vi "FPGA-no_chopper.vi"() -> ()   [LabVIEW 2009]
uses:
  Sequence.ctl
  Signal Options.ctl
  <vilib>/Platform/TimedLoop/XDataNode/XDataNode.xnode
  <vilib>/Platform/TimedLoop/XDataNode/loadlvalarms.vi
  <vilib>/Platform/TimedLoop/XDataNode/timing_clust.ctl
  <vilib>/Platform/TimedLoop/XDataNode/nitl_modes.ctl
  <vilib>/Platform/TimedLoop/XDataNode/wakeup.ctl
  <vilib>/eio/EIONode/EIONode.xnode
  <vilib>/rvi/eio/nirviEIOImplementation/nirviEIOImplementation.xnode
  <vilib>/rvi/eio/common/nirviEmuTemplateMethod_noerrors.vi
  <vilib>/rvi/eio/common/nirviEmuClasses.ctl
  <vilib>/Platform/TimedLoop/XDataNode/XDNodeRunTimeDep.lvlib
panel:
  in  "Squeezed AOM Signal 1+2 Sign":bool
  in  "Squeezed AOM Signal 2 start":u64
  in  "Squeezed AOM Signal 2 stop":u64
  in  "Trigger Phase Acquisition":bool
  in  "Phase Trigger Period":u32
  in  "Trigger Shot Aquisition":bool=TRUE
  in  "Shot Acquisiton Trigger Start":u64
  in  "Shot Acquisition Trigger Stop":u64
  in  "Memory Acquisition Trigger Stop":u64
  in  "WA Extra stop  6":u32
  in  "WA Extra start 6":u32
  in  "WA Extra stop  5":u32
  in  "WA Extra start 5":u32
  in  "WA Extra stop  4":u32
  in  "WA Extra start 4":u32
  in  "WA Extra stop  3":u32
  in  "WA Extra start 3":u32
  in  "WA Extra stop  2":u32
  in  "WA Extra start 2":u32
  in  "WA Extra start":u32
  in  "WA Extra stop":u32
  in  "WA Extra Sign":bool
  in  "WA Signal Switch 2 stop":u32
  in  "WA Signal Switch 2 start":u32
  in  "WA Signal Switch Sign":bool
  in  "WA Signal Switch stop":u32
  in  "WA Signal Switch start":u32
  in  "Squeezed AOM Signal Sign":bool
  in  "Squeezed AOM Control Sign":bool
  in  "Optical Density Sign":bool
  in  "SPME Gate 2 Sign":bool
  in  "SPME Gate 1 Sign":bool
  in  "SPME Signal Sign":bool
  in  "SPME Control Sign":bool
  in  "DLCZ Sign":bool
  in  "Raman Signal Sign":bool
  in  "Raman Control Sign":bool
  in  "Coherent Signal Sign":bool
  in  "WA Stop":bool
  in  "WA Trigger Output Sign":bool
  in  "WA Signal start":u32
  in  "WA Signal stop":u32
  in  "WA Signal Sign":bool
  in  "WA Repump start":u32
  in  "WA Repump stop":u32
  in  "WA Repump Sign":bool
  in  "WA Pump start":u32
  in  "WA Pump stop":u32
  in  "WA Pump Sign":bool
  in  "WA Control 2 - start":u32
  in  "WA Control 2 - stop":u32
  in  "WA Control 1 - start":u32
  in  "WA Control 1 - stop":u32
  in  "WA Control Sign":bool
  in  "WA Repetition Period":u32
  out "WA Active":bool
  in  "WA Trigger on Slope":enum8{"either", "false-true", "true-false"}(ring)=enum."true-false"
  out "WA Reset Interval":u64
  in  "WA Control Switch 2 - start":u32
  in  "WA Control Switch 2 - stop":u32
  in  "WA Control Switch 1 - start":u32
  in  "WA Control Switch 1 - stop":u32
  in  "WA Control Switch Sign":bool
  in  "Memory Acquisiton Trigger Start":u64
  in  "Memory Mode":bool
  out "Last N2":u64
  out "Last N1":u64
  in  "Desired Number of Trials":u64
  out "Number of Trials":u64
  out "Current N2":u64
  out "Current N1":u64
  in  "SPME Gate 2 - start":u64
  in  "SPME Gate 2 - stop":u64
  in  "SPME Gate 1 - start":u64
  in  "SPME Gate 1 - stop":u64
  out "SPME Count":u64
  out "Last SPME Interval between Resets":u64
  in  "SPME Period":u64
  in  "SPME Signal stop":u64
  in  "SPME Control - start":u64
  in  "Num of SPME Pulses per Mem Seq":u64=100
  in  "SPME Signal start":u64
  in  "SPME Control - stop":u64
  in  "SPME Start":u64
  in  "Raman/OD Acquisition Delay":u64
  in  "Squeezed AOM Signal 1 start":u64
  in  "Squeezed AOM Signal 1 stop":u64
  in  "Stop":bool
  out "Active":bool
  in  "Trapping Duration":u64
  in  "Pump Duration":u64
  in  "Repump Duration":u64
  out "Memory Timer":u64
  in  "Memory Mode":T1=enum."Coherent Memory Sequence"
  in  "Raman Control - stop":u64
  in  "Raman Control - start":u64
  in  "Raman Signal - stop":u64
  in  "Raman Signal - start":u64
  in  "Optical Density - start":u64
  in  "Optical Density - stop":u64
  in  "DLCZ width":u64
  in  "DLCZ Period":u32
  out "Last DLCZ Period":u64
  in  "DLCZ Stop":u64
  in  "DLCZ Start":u64
  in  "Control - start":u64
  in  "Control - stop":u64
  in  "Control Sign":bool
  out "Last Memory Period":u64
  in  "Coherent Signal start":u64
  in  "Coherent Signal stop":u64
  out "Global Time":u64
  in  "Output Trigger Sign":bool
  in  "Trigger on Slope":enum8{"either", "false-true", "true-false"}(ring)=enum."true-false"
  in  "Repetition Period":u32
  in  "Memory Sequence Duration":u64=240000
  out "Current State":T2
  out "Last Global Period":u64
  # "Alignment - Lights On"
  # "Corresponds to 5MHz by default"
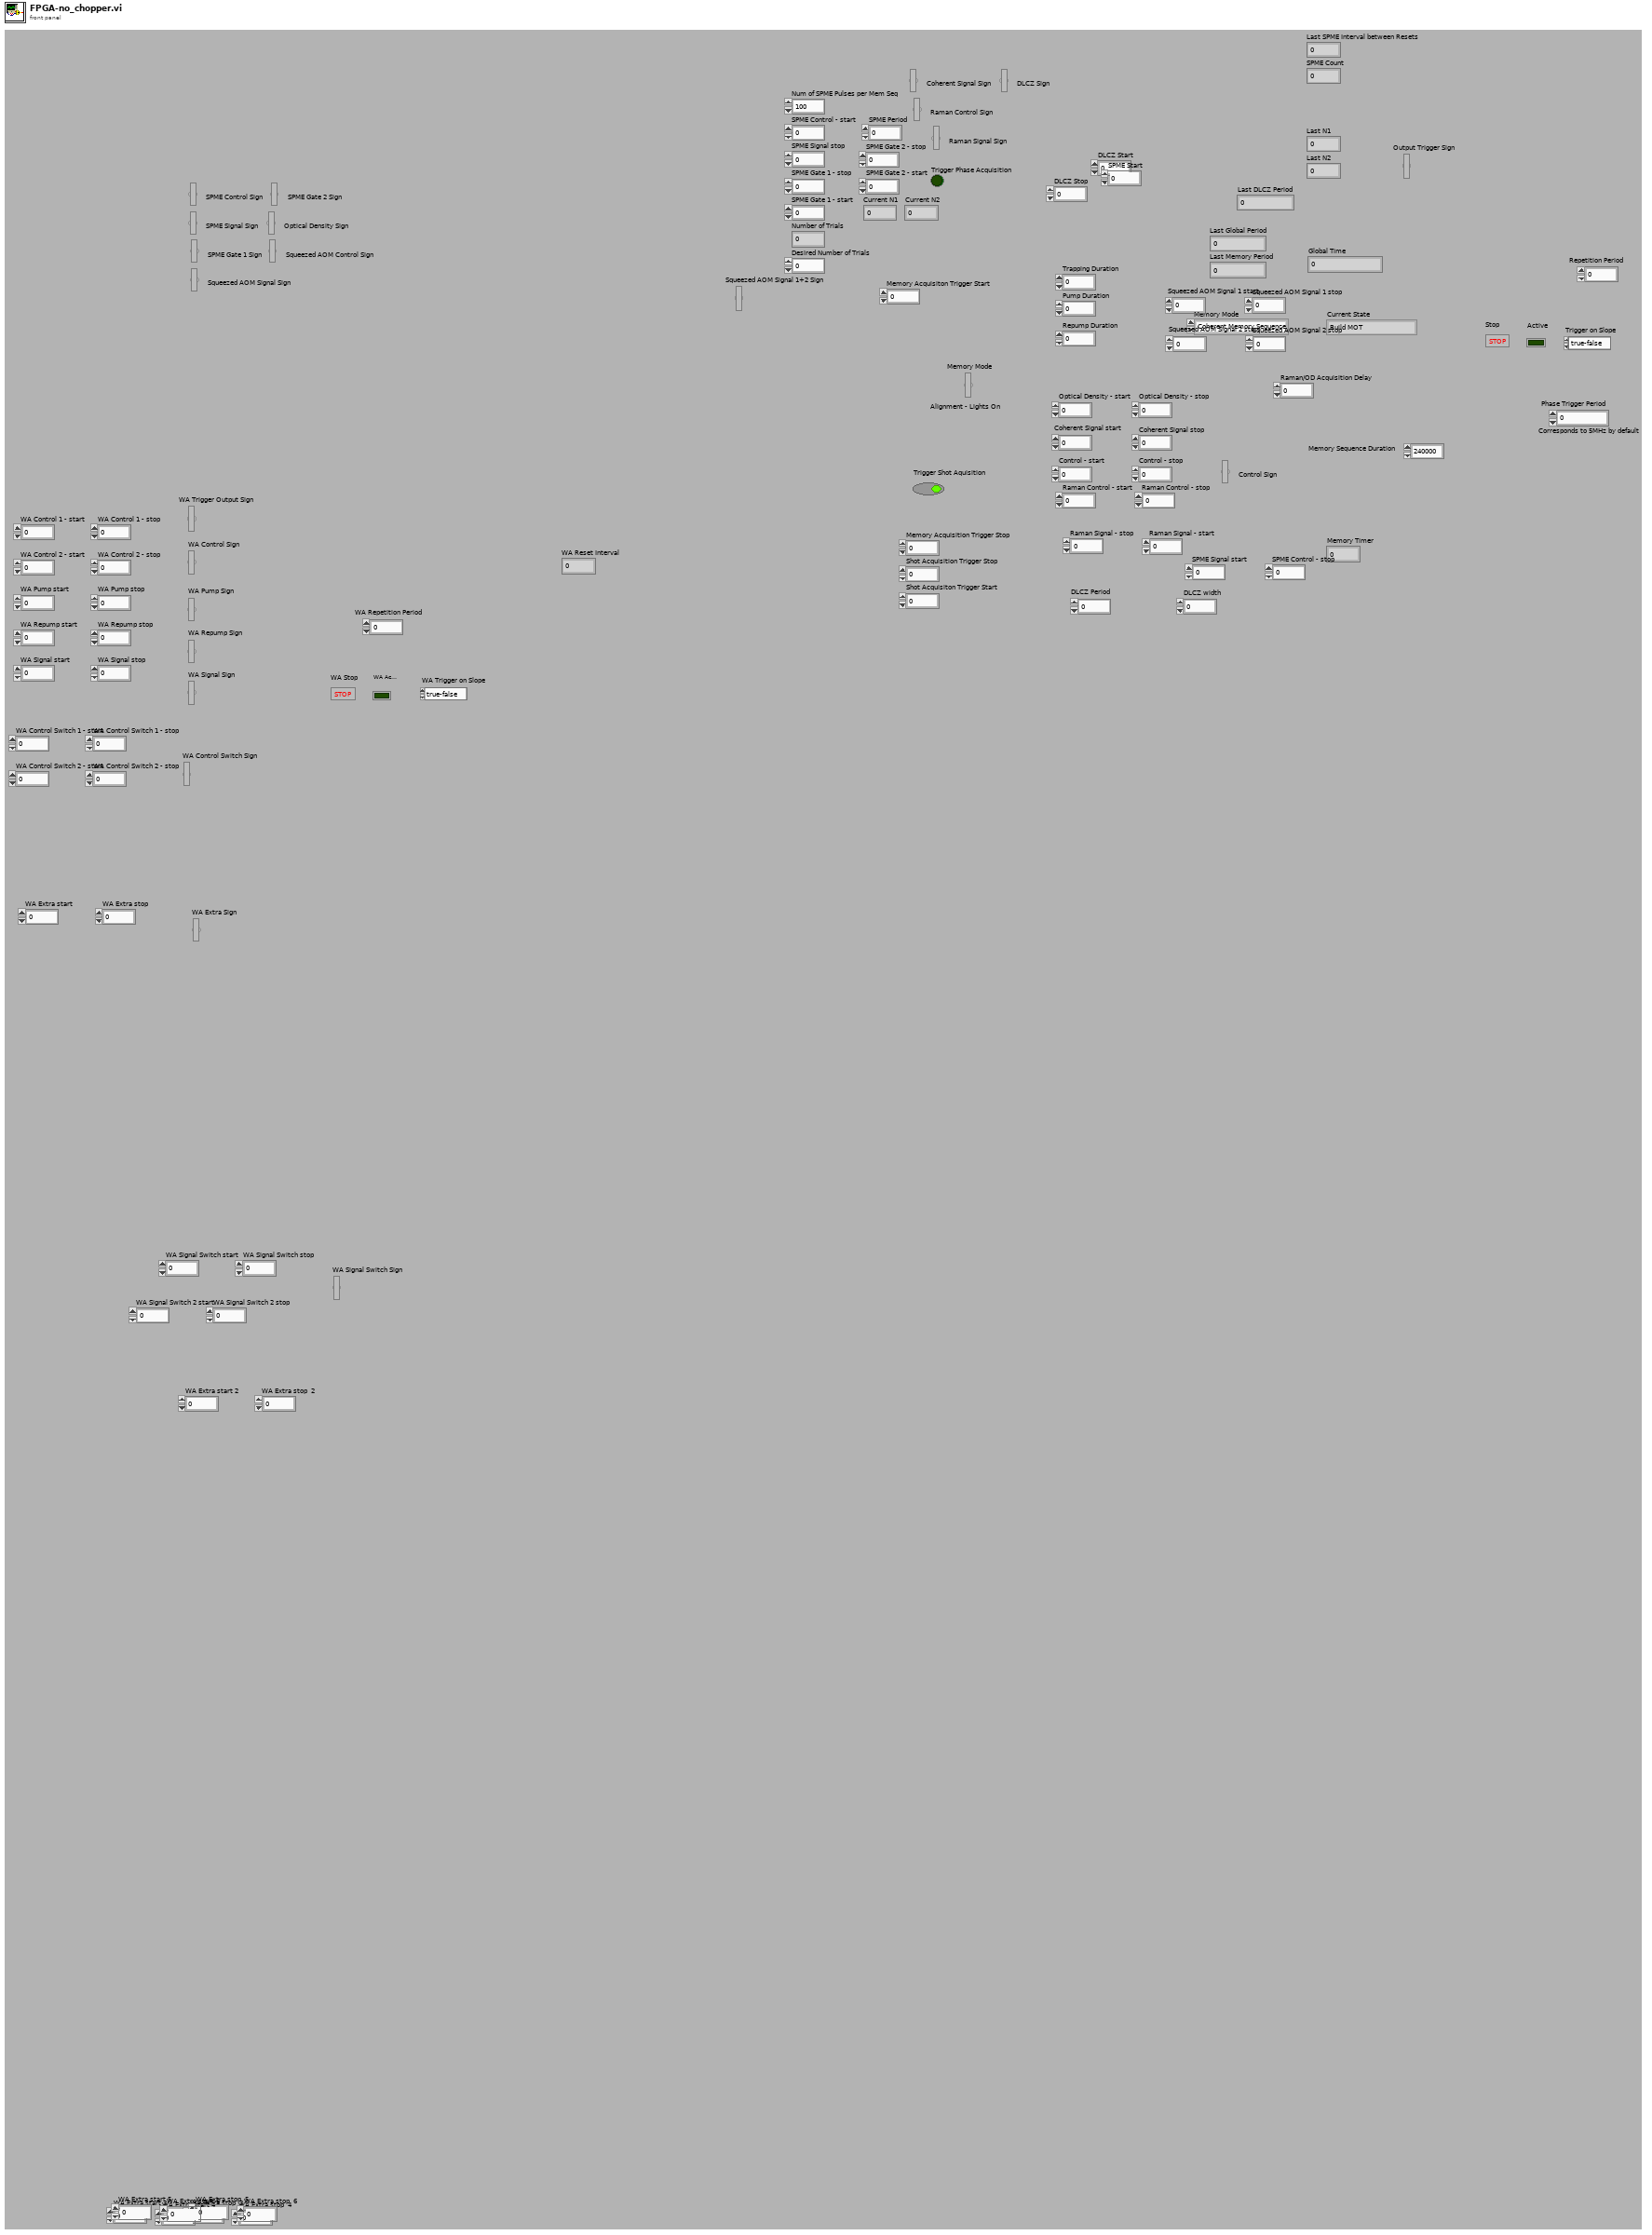
[diagram p1: front panel]
types:
  T1 = typedef "Signal Options.ctl" = enum16{"Cycle Trap - Standby", "Generate DLCZ Pulses", "Measure Optical Density", "Measure Raman", "Single Photon Memory Efficiency", "Coherent Memory Sequence", "Squeezed AOM Memory Sequence", "Squeezed Chopper Memory Sequence"}
  T2 = typedef "Sequence.ctl" = enum16{"Build MOT", "Memory Sequence", "Alignment - Lights On"}
  T3 = typedef "XDNodeRunTimeDep.lvlib/timing_clust.ctl" = cluster{"Expected End [f-1]":u64, "Actual End [f-1]":u64, "Finished Late? [f-1]":bool, "Expected End [i-1]":u64, "Actual End [i-1]":u64, "Finished Late? [i-1]":bool, "Expected Start [i]":u64, "Actual Start [i]":u64, "Expected Start [f]":u64, "Actual Start [f]":u64, "Source Name":string, "Structure Name":string, "Period":i64, "Deadline":i64, "Offset":i64, "Start":i64, "Priority":i32, "Timeout":i32, "Mode":T4, "Wakeup Reason":T5, "Error":errorcluster, "Source Type":string, "Secondary Source Type":string, "Global End Time":u64, "Global Start Time":u64, "Frame Duration":u64, "Iteration Duration":u64, "Assigned CPU":i32, "I/O Scan Engine Mode":u32}
  T4 = typedef "XDNodeRunTimeDep.lvlib/nitl_modes.ctl" = enum32{"No Change", "Process missed periods, maintain original phase", "Discard missed periods, maintain original phase", "Process missed periods, ignore original phase", "Discard missed periods, ignore original phase"}
  T5 = typedef "XDNodeRunTimeDep.lvlib/wakeup.ctl" = enum32{"Normal", "Aborted", "Asynchronous wakeup", "Timing source error", "Timed loop error", "Timeout"}
  T6 = typedef "nirviEmuClasses.ctl" = enum16{"IO Read", "IO Write", "Method", "Property Read", "Property Write"}
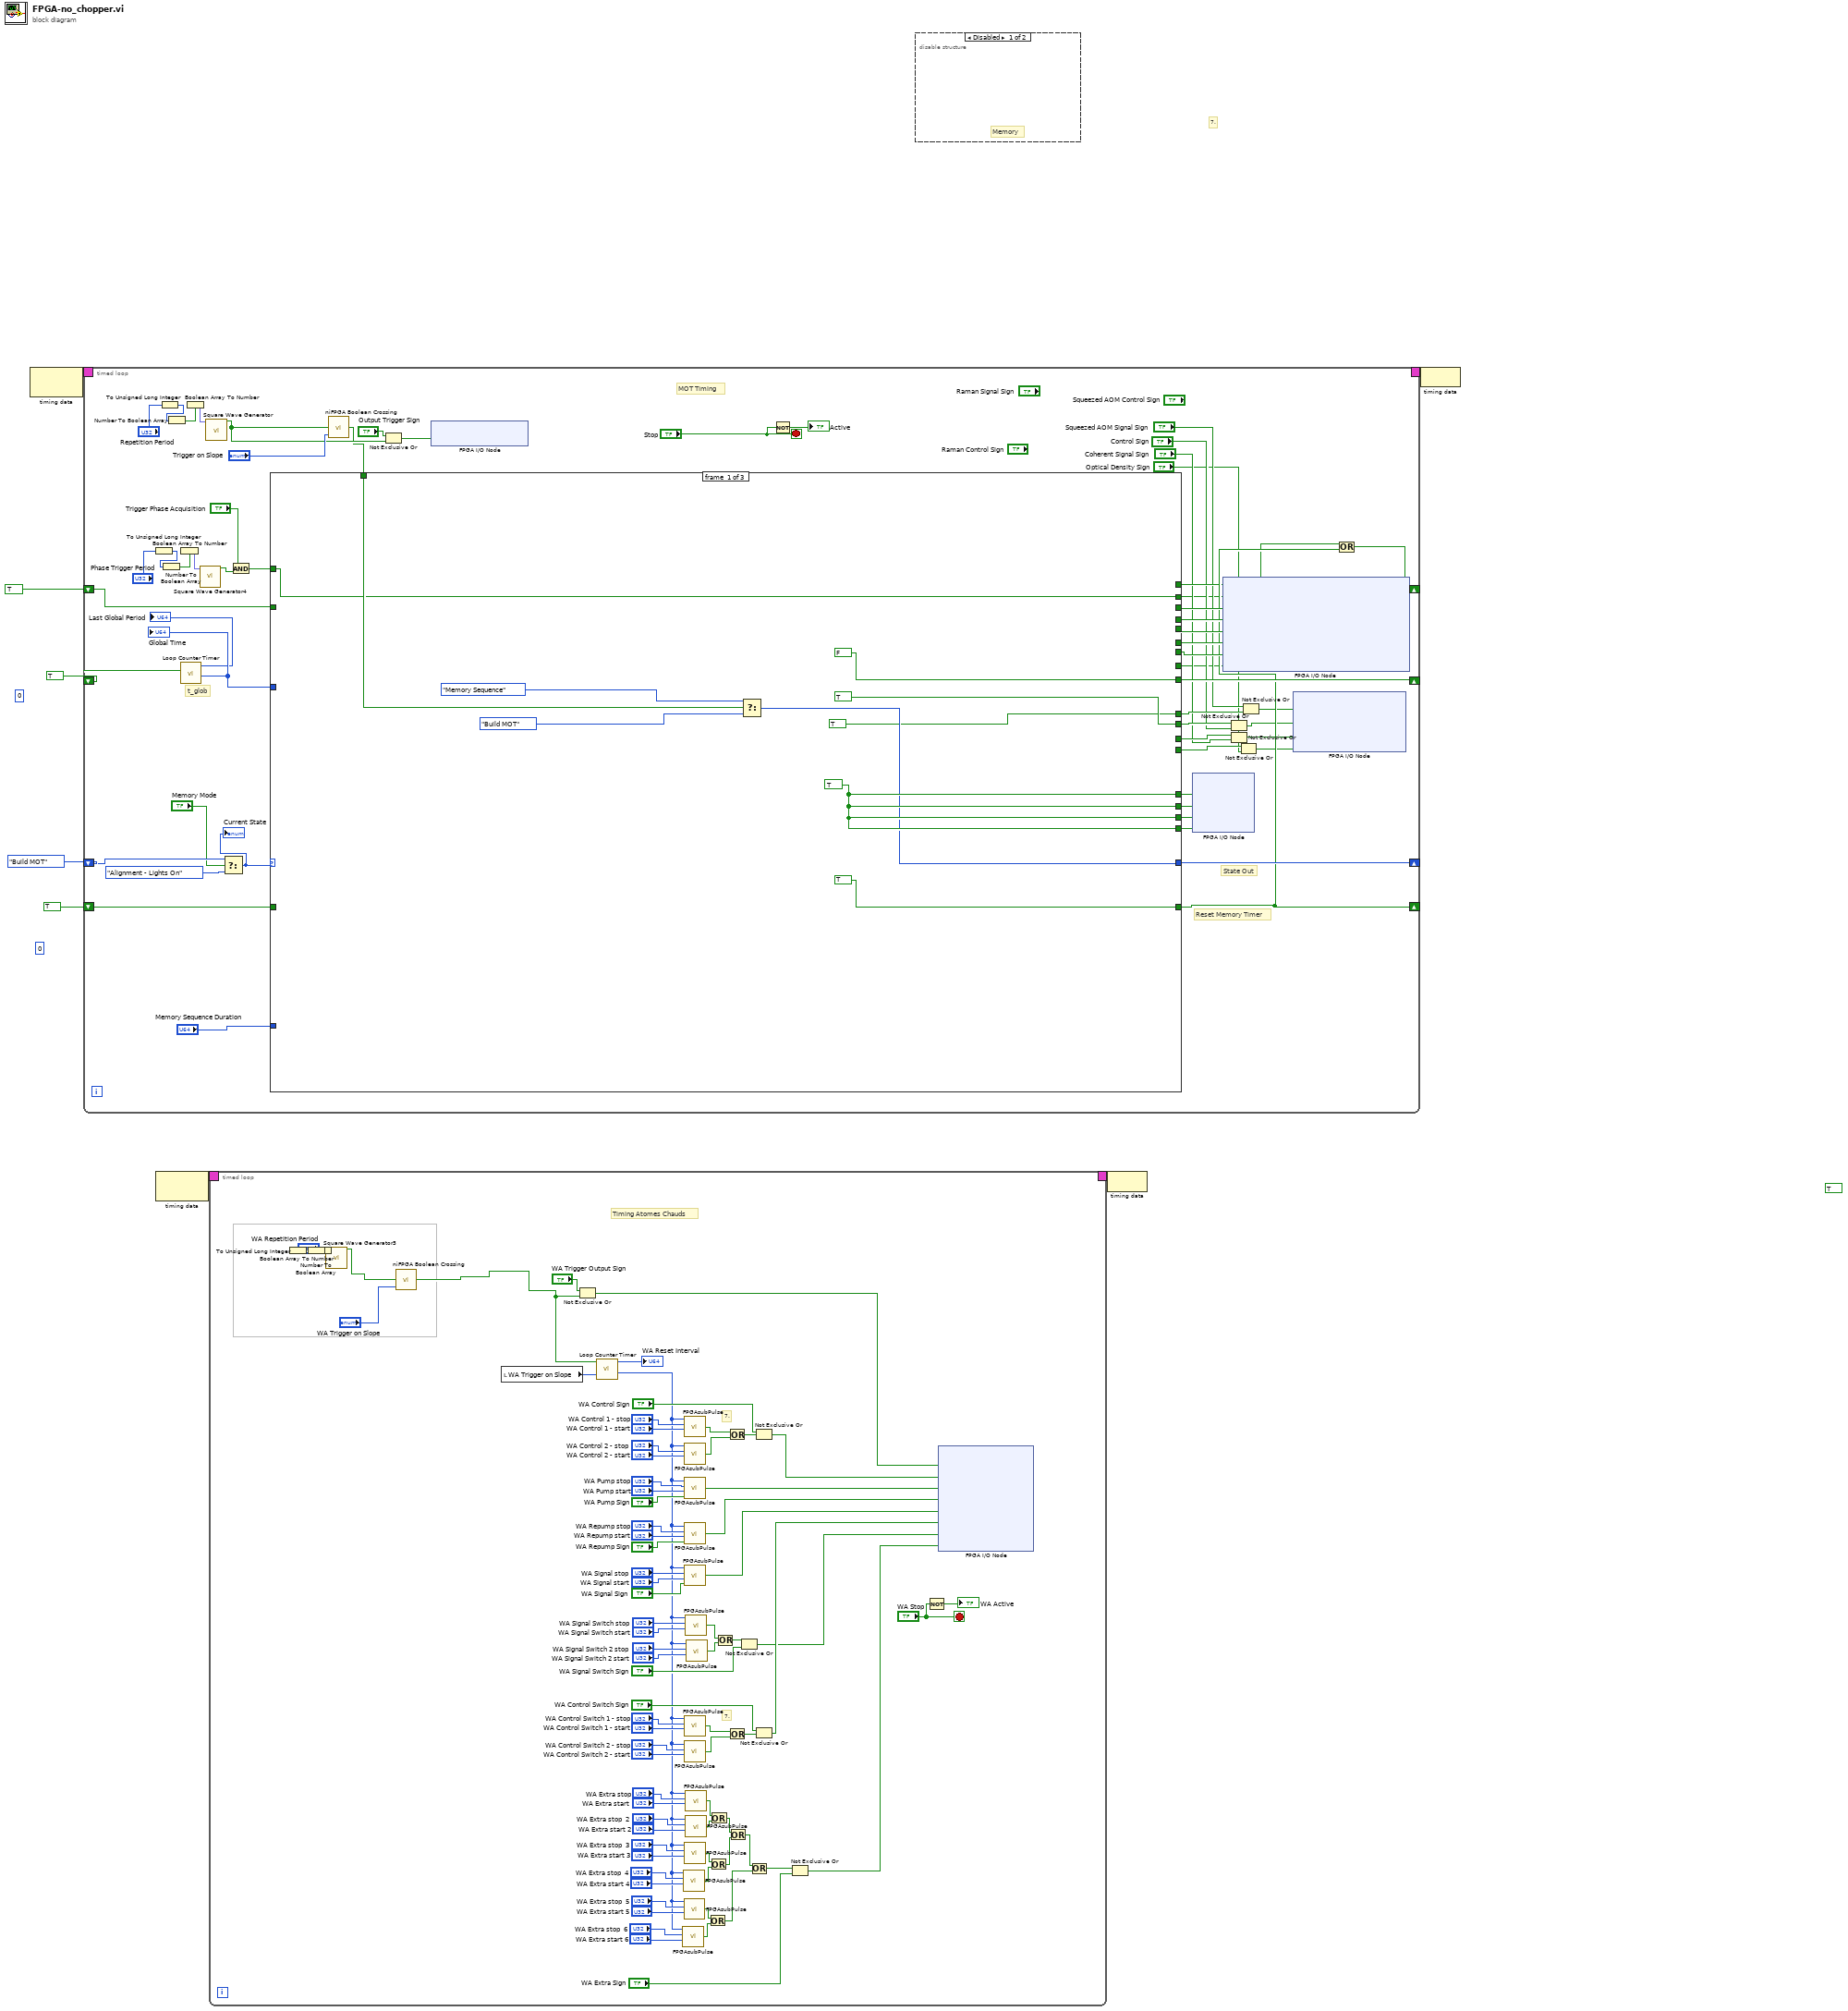
[diagram p0: block diagram]
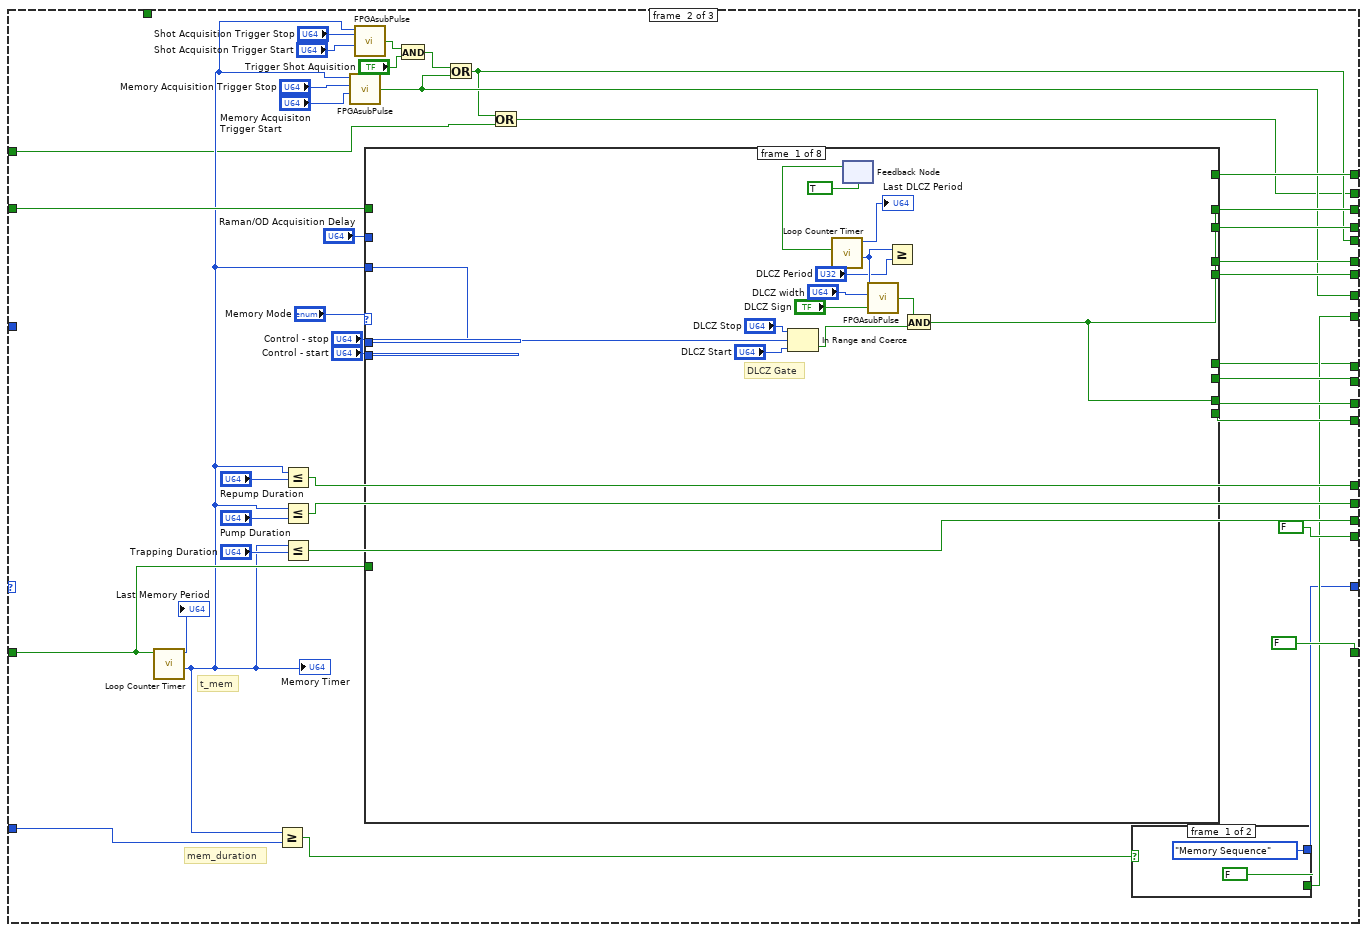
[diagram p3: hidden frame]
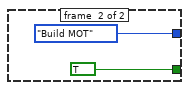
[diagram p4: hidden frame]
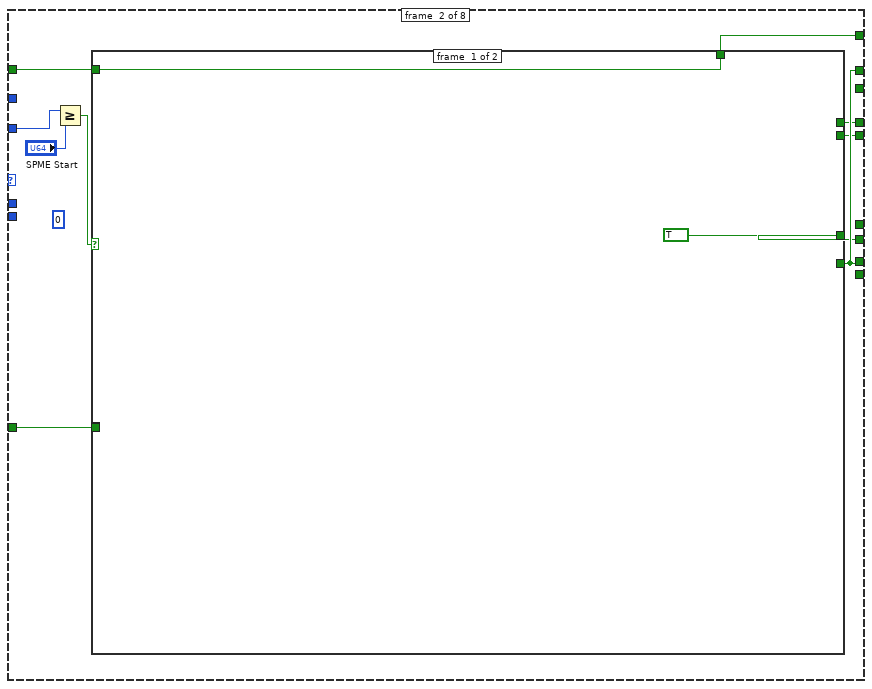
[diagram p5: hidden frame]
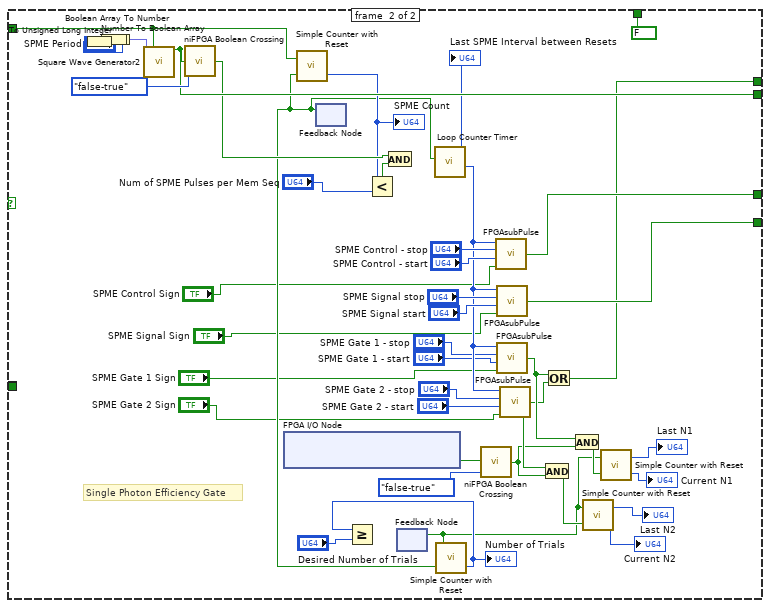
[diagram p6: hidden frame]
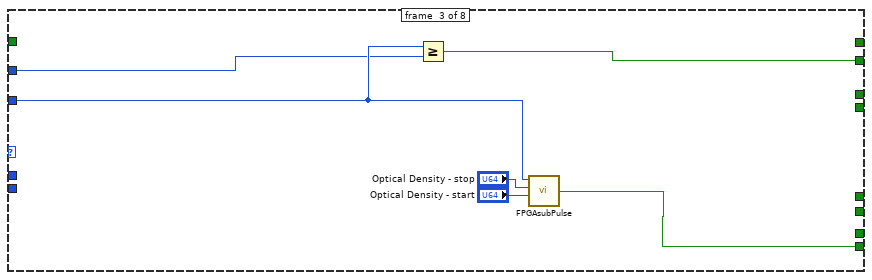
[diagram p7: hidden frame]
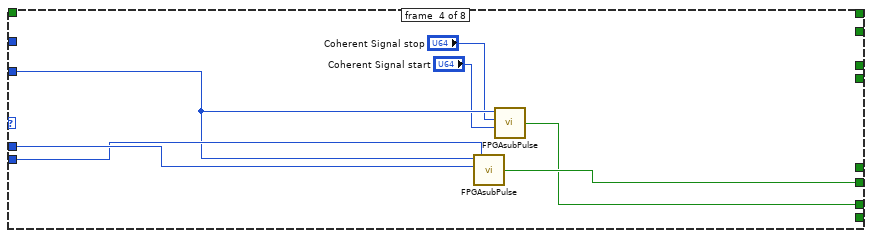
[diagram p8: hidden frame]
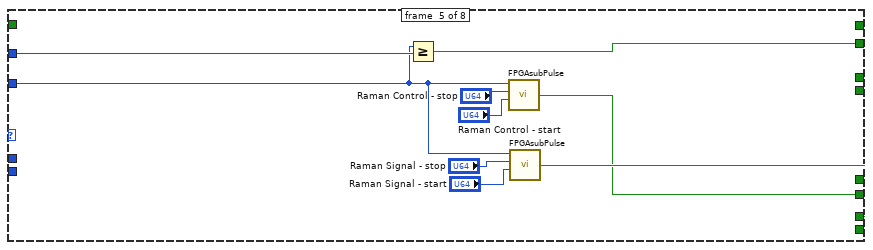
[diagram p9: hidden frame]
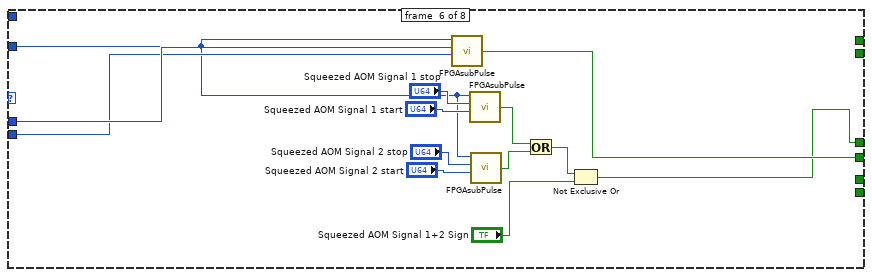
[diagram p10: hidden frame]
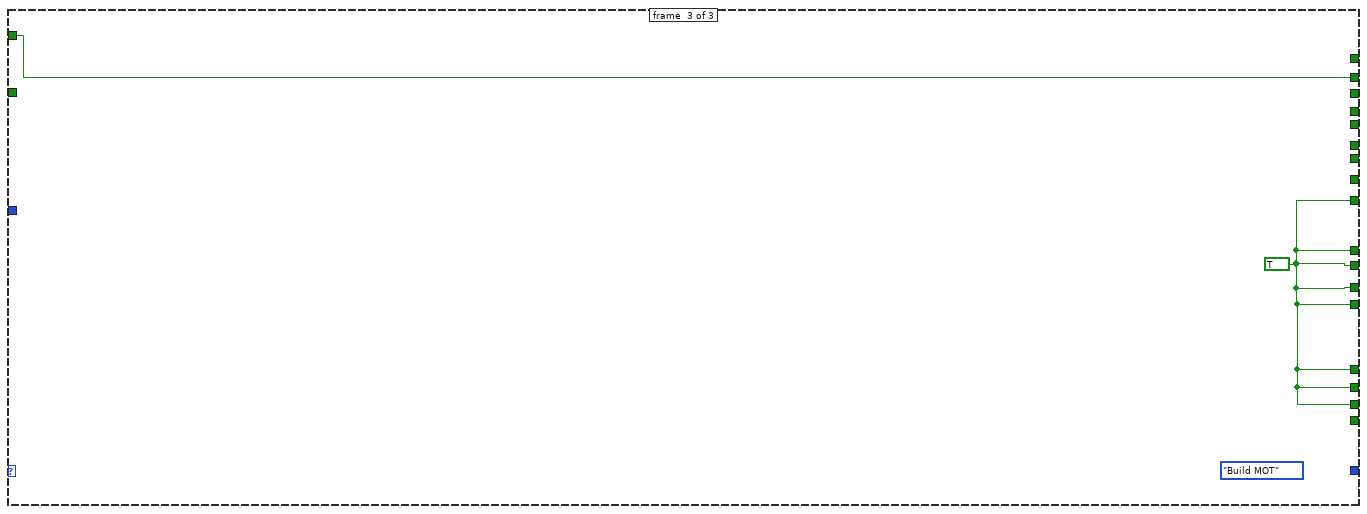
[diagram p13: hidden frame]
diagram:
  (unwired) u64 0
  (unwired) u64 0
  (unwired) TRUE
  # "7."
  n1 = node-c288() -> (w8:T3)  [unwired: 1 out]
  n2 = timed-loop {
    timing: w8 -> [_]
    timing-out: [_] -> w7
    shift-right: [w61] -> _
    shift-left: Sequence."Build MOT" ("Sequence") -> [w29]
    shift-right: [w43] -> _
    shift-left: TRUE -> [w54]
    shift-right: [w33] -> _
    shift-left: TRUE -> [w49]
    shift-right: [w31] -> _
    shift-left: TRUE -> [w32]
    stop <- "Stop" stop-if-true
    # "MOT Timing"
    # "Reset Memory Timer"
    # "State Out"
    # "t_glob"
    n3 = To Unsigned Long Integer(number="Phase Trigger Period") -> (unsigned 32bit integer=w12:u32)
    n4 = To Unsigned Long Integer(number="Repetition Period") -> (unsigned 32bit integer=w55:u32)
    n5 = Number To Boolean Array(number=w12) -> (Boolean array=w14:bool[])
    n6 = Number To Boolean Array(number=w55) -> (Boolean array=w57:bool[])
    n7 = Boolean Array To Number(Boolean array=w14) -> (number=w13:fxp<+,32,0>)
    n8 = call "Loop Counter Timer.vi"("Reset"=w54) -> ("Loop Counter"=w53:u64, "Last Interval between Resets"=→"Last Global Period":u64)  [unwired: 3 in, 2 out]
    "Global Time" <- w53
    n9 = Boolean Array To Number(Boolean array=w57) -> (number=w56:fxp<+,32,0>)
    n10 = call "Square Wave Generator4"("frequency (periods/tick)"=w13) -> ("square wave out"=w11:bool)  [unwired: 14 in]
    n11 = call "Square Wave Generator"("frequency (periods/tick)"=w56) -> ("square wave out"=w39:bool)  [unwired: 14 in]
    n12 = Select(t=w29, s="Memory Mode", f=Sequence."Alignment - Lights On" ("Sequence")) -> (s? t:f=w27:T2)
    "Current State" <- w27
    n13 = And(x="Trigger Phase Acquisition", y=w11) -> (x .and. y?=w9:bool)
    n14 = call <vilib>:"niFPGA Boolean Crossing.vi"("input"=w39, "direction"="Trigger on Slope") -> ("crossing"=w37:bool)  [unwired: 1 in, 6 out]
    n15 = case shown="\"Memory Sequence\"" w27 {
      tunnel: [w246 w272 _] -> w61
      tunnel: [w247 FALSE _] -> w62
      tunnel: [FALSE w273 w423] -> w43
      tunnel: w53 -> [_ _ _]
      tunnel: [w247 w283 w423] -> w52
      tunnel: [w247 w284 w423] -> w51
      tunnel: [w247 w285 w423] -> w50
      tunnel: [TRUE FALSE _] -> w33
      tunnel: w49 -> [_ w265 _]
      tunnel: "Memory Sequence Duration" -> [_ w289 _]
      tunnel: [TRUE ("Boolean") w281 w423] -> w47
      tunnel: [_ w280 w423] -> w46
      tunnel: [_ w279 w423] -> w45
      tunnel: [_ w271 _] -> w42
      tunnel: [_ w269 _] -> w41
      tunnel: [TRUE ("Boolean") w270 w423] -> w40
      tunnel: w37 -> [w245 _ _]
      tunnel: [_ w253 _] -> w36
      tunnel: [_ w267 _] -> w35
      tunnel: [_ w266 _] -> w34
      tunnel: w32 -> [_ w264 _]
      tunnel: [_ w263 _] -> w30
      tunnel: [_ w254 _] -> w17
      tunnel: [w241 w252 w422] -> w16
      tunnel: w9 -> [w241 w251 w422]
      frame #0 {
        w247 = TRUE
        n16 = Select(t=Sequence."Memory Sequence" ("Sequence"), s=w245, f=Sequence."Build MOT" ("Sequence")) -> (s? t:f=w246:T2)
      }
      frame #1 {
        # "mem_duration"
        # "t_mem"
        n17 = call "Loop Counter Timer.vi"("Reset"=w265) -> ("Loop Counter"=w258:u64, "Last Interval between Resets"=→"Last Memory Period":u64)  [unwired: 3 in, 2 out]
        "Memory Timer" <- w258
        n18 = Greater Or Equal?(x=w258, y=w289) -> (x >= y?=w274:bool)
        n19 = Less Or Equal?(x=w258, y="Repump Duration") -> (x <= y?=w283:bool)
        n20 = Less Or Equal?(x=w258, y="Pump Duration") -> (x <= y?=w284:bool)
        n21 = Less Or Equal?(x=w258, y="Trapping Duration") -> (x <= y?=w285:bool)
        n22 = call "FPGAsubPulse.vi"("Signal start"="Memory Acquisiton Trigger Start", "Signal stop"="Memory Acquisition Trigger Stop", "Clock"=w258) -> ("Boolean"=w254:bool)  [unwired: 1 in]
        n23 = call "FPGAsubPulse.vi"("Signal start"="Shot Acquisiton Trigger Start", "Signal stop"="Shot Acquisition Trigger Stop", "Clock"=w258) -> ("Boolean"=w257:bool)  [unwired: 1 in]
        n24 = case shown="\"Squeezed AOM Memory Sequence\"" "Memory Mode" {
          tunnel: w258 -> [w300 w318 w389 w397 w401 w414 _ _]
          tunnel: [_ w314 _ w396 w403 w419 _ _] -> w281
          tunnel: [_ _ w390 _ _ _ _ _] -> w280
          tunnel: [w296 w315 _ w395 w408 _ _ _] -> w279
          tunnel: "Control - stop" -> [_ _ _ w399 _ w421 _ _]
          tunnel: "Control - start" -> [_ _ _ w398 _ w420 _ _]
          tunnel: [_ _ w387 _ w400 _ _ _] -> w271
          tunnel: [w296 w315 _ _ _ _ _ _] -> w269
          tunnel: [_ _ _ _ _ w410 _ _] -> w270
          tunnel: "Raman/OD Acquisition Delay" -> [_ _ w388 _ w402 _ _ _]
          tunnel: [_ w313 _ _ _ _ _ _] -> w267
          tunnel: [_ w312 _ _ _ _ _ _] -> w266
          tunnel: w265 -> [_ w311 _ _ _ _ _ _]
          tunnel: w264 -> [_ w310 _ _ _ _ _ _]
          tunnel: [_ w309 _ _ _ _ _ _] -> w263
          frame #0 {
            # "DLCZ Gate"
            n25 = In Range and Coerce(upper limit="DLCZ Stop", x=w300, lower limit="DLCZ Start") -> (In Range?=w301:bool)  [unwired: 1 out]
            n26 = feedback #1(TRUE) -> (w306:bool)
            n27 = call "Loop Counter Timer.vi"("Reset"=w306) -> ("Loop Counter"=w304:u64, "Last Interval between Resets"=→"Last DLCZ Period":u64)  [unwired: 3 in, 2 out]
            n28 = call "FPGAsubPulse.vi"("Signal Sign"="DLCZ Sign", "Signal stop"="DLCZ width", "Clock"=w304) -> ("Boolean"=w297:bool)  [unwired: 1 in]
            n29 = Greater Or Equal?(x=w304, y="DLCZ Period") -> (x >= y?=w307:bool)
            n30 = And(x=w297, y=w301) -> (x .and. y?=w296:bool)
          }
          frame #1 {
            (unwired) u64 0
            n31 = Greater Or Equal?(x=w318, y="SPME Start") -> (x >= y?=w316:bool)
            n32 = case shown="False" w316 {
              tunnel: [_ w352] -> w315
              tunnel: [TRUE ("Boolean") w367] -> w314
              tunnel: [_ w356] -> w313
              tunnel: [_ w346] -> w312
              tunnel: [_ w355] -> _
              tunnel: w311 -> [_ w355]
              tunnel: w310 -> [w319 w331]
              tunnel: [w319 FALSE] -> w309
              frame #0 {
              }
              frame #1 {
                # "Single Photon Efficiency Gate"
                n33 = To Unsigned Long Integer(number="SPME Period") -> (unsigned 32bit integer=w365:u32)
                n34 = Number To Boolean Array(number=w365) -> (Boolean array=w364:bool[])
                n35 = Boolean Array To Number(Boolean array=w364) -> (number=w363:fxp<+,32,0>)
                n36 = call "Square Wave Generator2"("frequency (periods/tick)"=w363, "reset"=w331) -> ("square wave out"=w356:bool)  [unwired: 13 in]
                n37 = call <vilib>:"niFPGA Boolean Crossing.vi"("input"=w356, "direction"=enum8{"either", "false-true", "true-false"}."false-true") -> ("crossing"=w332:bool)  [unwired: 1 in, 6 out]
                n38 = xnode "FPGA I/O Node"() -> ("SPME APD Counter Input"=w339:bool)  [unwired: 1 in, 1 out]
                n39 = feedback #2() -> (w328:bool)  [unwired: 1 in]
                n40 = call "Simple Counter with Reset.vi"("Add"=w328, "Reset"=w331) -> ("Loop Counter"=w330:u64)  [unwired: 1 out]
                "SPME Count" <- w330
                n41 = Less?(x=w330, y="Num of SPME Pulses per Mem Seq") -> (x < y?=w361:bool)
                n42 = And(x=w332, y=w361) -> (x .and. y?=w329:bool)
                n43 = feedback #3() -> (w333:bool)  [unwired: 1 in]
                n44 = call "Loop Counter Timer.vi"("Reset"=w328) -> ("Loop Counter"=w351:u64, "Last Interval between Resets"=→"Last SPME Interval between Resets":u64)  [unwired: 3 in, 2 out]
                n45 = call "Simple Counter with Reset.vi"("Add"=w328, "Reset"=w333) -> ("Loop Counter"=w341:u64)  [unwired: 1 out]
                "Number of Trials" <- w341
                n46 = Greater Or Equal?(x=w341, y="Desired Number of Trials") -> (x >= y?=w340:bool)
                n47 = call <vilib>:"niFPGA Boolean Crossing.vi"("input"=w339, "direction"=enum8{"either", "false-true", "true-false"}."false-true") -> ("crossing"=w338:bool)  [unwired: 1 in, 6 out]
                n48 = call "FPGAsubPulse.vi"("Signal Sign"="SPME Control Sign", "Signal start"="SPME Control - start", "Signal stop"="SPME Control - stop", "Clock"=w351) -> ("Boolean"=w367:bool)
                n49 = call "FPGAsubPulse.vi"("Signal Sign"="SPME Signal Sign", "Signal start"="SPME Signal start", "Signal stop"="SPME Signal stop", "Clock"=w351) -> ("Boolean"=w352:bool)
                n50 = call "FPGAsubPulse.vi"("Signal Sign"="SPME Gate 1 Sign", "Signal start"="SPME Gate 1 - start", "Signal stop"="SPME Gate 1 - stop", "Clock"=w351) -> ("Boolean"=w343:bool)
                n51 = call "FPGAsubPulse.vi"("Signal Sign"="SPME Gate 2 Sign", "Signal start"="SPME Gate 2 - start", "Signal stop"="SPME Gate 2 - stop", "Clock"=w351) -> ("Boolean"=w342:bool)
                n52 = And(x=w342, y=w338) -> (x .and. y?=w336:bool)
                n53 = Or(x=w343, y=w342) -> (x .or. y?=w346:bool)
                n54 = And(x=w343, y=w338) -> (x .and. y?=w335:bool)
                n55 = call "Simple Counter with Reset.vi"("Add"=w336, "Reset"=w333) -> ("Loop Counter"=→"Current N2":u64, "Last Count Before Reset"=→"Last N2":u64)
                n56 = call "Simple Counter with Reset.vi"("Add"=w335, "Reset"=w333) -> ("Loop Counter"=→"Current N1":u64, "Last Count Before Reset"=→"Last N1":u64)
              }
            }
          }
          frame #2 {
            n57 = Greater Or Equal?(x=w389, y=w388) -> (x >= y?=w387:bool)
            n58 = call "FPGAsubPulse.vi"("Signal start"="Optical Density - start", "Signal stop"="Optical Density - stop", "Clock"=w389) -> ("Boolean"=w390:bool)  [unwired: 1 in]
          }
          frame #3 {
            n59 = call "FPGAsubPulse.vi"("Signal start"=w398, "Signal stop"=w399, "Clock"=w397) -> ("Boolean"=w396:bool)  [unwired: 1 in]
            n60 = call "FPGAsubPulse.vi"("Signal start"="Coherent Signal start", "Signal stop"="Coherent Signal stop", "Clock"=w397) -> ("Boolean"=w395:bool)  [unwired: 1 in]
          }
          frame #4 {
            n61 = Greater Or Equal?(x=w401, y=w402) -> (x >= y?=w400:bool)
            n62 = call "FPGAsubPulse.vi"("Signal start"="Raman Control - start", "Signal stop"="Raman Control - stop", "Clock"=w401) -> ("Boolean"=w403:bool)  [unwired: 1 in]
            n63 = call "FPGAsubPulse.vi"("Signal start"="Raman Signal - start", "Signal stop"="Raman Signal - stop", "Clock"=w401) -> ("Boolean"=w408:bool)  [unwired: 1 in]
          }
          frame #5 {
            n64 = call "FPGAsubPulse.vi"("Signal start"=w420, "Signal stop"=w421, "Clock"=w414) -> ("Boolean"=w419:bool)  [unwired: 1 in]
            n65 = call "FPGAsubPulse.vi"("Signal start"="Squeezed AOM Signal 1 start", "Signal stop"="Squeezed AOM Signal 1 stop", "Clock"=w414) -> ("Boolean"=w412:bool)  [unwired: 1 in]
            n66 = call "FPGAsubPulse.vi"("Signal start"="Squeezed AOM Signal 2 start", "Signal stop"="Squeezed AOM Signal 2 stop", "Clock"=w414) -> ("Boolean"=w413:bool)  [unwired: 1 in]
            n67 = Or(x=w412, y=w413) -> (x .or. y?=w411:bool)
            n68 = Not Exclusive Or(1:"Squeezed AOM Signal 1+2 Sign", 2:w411) -> (0:w410:bool)
          }
          frame #6 {
          }
          frame #7 {
          }
        }
        n69 = And(x=w257, y="Trigger Shot Aquisition") -> (x .and. y?=w256:bool)
        n70 = Or(x=w256, y=w254) -> (x .or. y?=w253:bool)
        n71 = Or(x=w253, y=w251) -> (x .or. y?=w252:bool)
        n72 = case shown="True" w274 {
          tunnel: [FALSE TRUE] -> w273
          tunnel: [Sequence."Memory Sequence" ("Sequence") Sequence."Build MOT" ("Sequence")] -> w272
          frame #0 {
          }
          frame #1 {
          }
        }
      }
      frame #2 {
        (unwired) Sequence."Build MOT" ("Sequence")
        w423 = TRUE ("Boolean")
      }
    }
    n73 = Not Exclusive Or(1:w39, 2:"Output Trigger Sign") -> (0:w38:bool)
    n74 = xnode "FPGA I/O Node"("Experiment Trigger"=w38) -> ()  [unwired: 1 in, 1 out]
    n75 = Not(x="Stop") -> (.not. x?=→"Active":bool)
    n76 = xnode "FPGA I/O Node"("Repump"=w52, "Pump"=w51, "Trapping"=w50, "B-Field"=w62) -> ()  [unwired: 4 in, 4 out]
    n77 = xnode "FPGA I/O Node"("Memory-Shot-Phase Acquisition Trigger"=w16, "APD1 Gate"=w41, "Raman/Optical Density Acquisition Trigger"=w42, "Memory-Shot Aquisition Trigger"=w36, "Single Photon Memory Gate"=w34, "SPME Timer"=w35, "Memory Only Acquisition Trigger  for Phase"=w17) -> ()  [unwired: 7 in, 7 out]
    n78 = Not Exclusive Or(1:"Control Sign", 2:w47) -> (0:w23:bool)
    n79 = Not Exclusive Or(1:"Coherent Signal Sign", 2:w45) -> (0:w21:bool)
    n80 = Not Exclusive Or(1:"Optical Density Sign", 2:w46) -> (0:w19:bool)
    n81 = Not Exclusive Or(1:w40, 2:"Squeezed AOM Signal Sign") -> (0:w25:bool)
    n82 = xnode "FPGA I/O Node"("Pulsed Squeezing AOM"=w25, "Control"=w23, "Signal"=w21, "Optical Density"=w19) -> ()  [unwired: 4 in, 4 out]
    n83 = Or(x=w30, y=w33) -> (x .or. y?=w31:bool)
  }
  n84 = node-c288() -> (w2:T3)  [unwired: 1 out]
  n85 = timed-loop {
    timing: w2 -> [_]
    timing-out: [_] -> w1
    stop <- "WA Stop" stop-if-true
    # "Timing Atomes Chauds"
    # "7."
    # "7."
    n86 = To Unsigned Long Integer(number="WA Repetition Period") -> (unsigned 32bit integer=w465:u32)
    n87 = Number To Boolean Array(number=w465) -> (Boolean array=w463:bool[])
    n88 = Boolean Array To Number(Boolean array=w463) -> (number=w464:fxp<+,32,0>)
    n89 = call "Square Wave Generator3"("frequency (periods/tick)"=w464) -> ("square wave out"=w461:bool)  [unwired: 14 in]
    n90 = call <vilib>:"niFPGA Boolean Crossing.vi"("input"=w461, "direction"="WA Trigger on Slope") -> ("crossing"=w462:bool)  [unwired: 1 in, 6 out]
    n91 = local read "WA Trigger on Slope"() -> (w480:enum8{"either", "false-true", "true-false"})
    n92 = Not Exclusive Or(1:w462, 2:"WA Trigger Output Sign") -> (0:w479:bool)
    n93 = call "Loop Counter Timer.vi"("Trigger Direction"=w480, "Waveform"=w462) -> ("Loop Counter"=w429:u64, "Last Interval between Resets"=→"WA Reset Interval":u64)  [unwired: 2 in, 2 out]
    n94 = call "FPGAsubPulse.vi"("Signal start"="WA Extra start 6", "Signal stop"="WA Extra stop  6", "Clock"=w429) -> ("Boolean"=w430:bool)  [unwired: 1 in]
    n95 = call "FPGAsubPulse.vi"("Signal start"="WA Extra start 4", "Signal stop"="WA Extra stop  4", "Clock"=w429) -> ("Boolean"=w436:bool)  [unwired: 1 in]
    n96 = call "FPGAsubPulse.vi"("Signal start"="WA Extra start 5", "Signal stop"="WA Extra stop  5", "Clock"=w429) -> ("Boolean"=w431:bool)  [unwired: 1 in]
    n97 = call "FPGAsubPulse.vi"("Signal start"="WA Control 1 - start", "Signal stop"="WA Control 1 - stop", "Clock"=w429) -> ("Boolean"=w489:bool)  [unwired: 1 in]
    n98 = call "FPGAsubPulse.vi"("Signal start"="WA Control 2 - start", "Signal stop"="WA Control 2 - stop", "Clock"=w429) -> ("Boolean"=w488:bool)  [unwired: 1 in]
    n99 = call "FPGAsubPulse.vi"("Signal Sign"="WA Pump Sign", "Signal start"="WA Pump start", "Signal stop"="WA Pump stop", "Clock"=w429) -> ("Boolean"=w477:bool)
    n100 = call "FPGAsubPulse.vi"("Signal Sign"="WA Repump Sign", "Signal start"="WA Repump start", "Signal stop"="WA Repump stop", "Clock"=w429) -> ("Boolean"=w476:bool)
    n101 = call "FPGAsubPulse.vi"("Signal Sign"="WA Signal Sign", "Signal start"="WA Signal start", "Signal stop"="WA Signal stop", "Clock"=w429) -> ("Boolean"=w475:bool)
    n102 = call "FPGAsubPulse.vi"("Signal start"="WA Control Switch 1 - start", "Signal stop"="WA Control Switch 1 - stop", "Clock"=w429) -> ("Boolean"=w471:bool)  [unwired: 1 in]
    n103 = call "FPGAsubPulse.vi"("Signal start"="WA Control Switch 2 - start", "Signal stop"="WA Control Switch 2 - stop", "Clock"=w429) -> ("Boolean"=w472:bool)  [unwired: 1 in]
    n104 = call "FPGAsubPulse.vi"("Signal start"="WA Extra start 3", "Signal stop"="WA Extra stop  3", "Clock"=w429) -> ("Boolean"=w439:bool)  [unwired: 1 in]
    n105 = call "FPGAsubPulse.vi"("Signal start"="WA Signal Switch start", "Signal stop"="WA Signal Switch stop", "Clock"=w429) -> ("Boolean"=w456:bool)  [unwired: 1 in]
    n106 = call "FPGAsubPulse.vi"("Signal start"="WA Extra start", "Signal stop"="WA Extra stop", "Clock"=w429) -> ("Boolean"=w447:bool)  [unwired: 1 in]
    n107 = call "FPGAsubPulse.vi"("Signal start"="WA Extra start 2", "Signal stop"="WA Extra stop  2", "Clock"=w429) -> ("Boolean"=w446:bool)  [unwired: 1 in]
    n108 = call "FPGAsubPulse.vi"("Signal start"="WA Signal Switch 2 start", "Signal stop"="WA Signal Switch 2 stop", "Clock"=w429) -> ("Boolean"=w455:bool)  [unwired: 1 in]
    n109 = Or(x=w431, y=w430) -> (x .or. y?=w427:bool)
    n110 = Or(x=w439, y=w436) -> (x .or. y?=w438:bool)
    n111 = Or(x=w447, y=w446) -> (x .or. y?=w437:bool)
    n112 = Or(x=w456, y=w455) -> (x .or. y?=w452:bool)
    n113 = Or(x=w489, y=w488) -> (x .or. y?=w484:bool)
    n114 = Or(x=w471, y=w472) -> (x .or. y?=w473:bool)
    n115 = Or(x=w437, y=w438) -> (x .or. y?=w428:bool)
    n116 = Not Exclusive Or(1:"WA Signal Switch Sign", 2:w452) -> (0:w451:bool)
    n117 = Or(x=w428, y=w427) -> (x .or. y?=w426:bool)
    n118 = Not Exclusive Or(1:w484, 2:"WA Control Sign") -> (0:w478:bool)
    n119 = Not Exclusive Or(1:w473, 2:"WA Control Switch Sign") -> (0:w466:bool)
    n120 = Not Exclusive Or(1:"WA Extra Sign", 2:w426) -> (0:w444:bool)
    n121 = Not(x="WA Stop") -> (.not. x?=→"WA Active":bool)
    n122 = xnode "FPGA I/O Node"("WA trigger"=w479, "WA control"=w478, "WA pump"=w477, "WA repump"=w476, "WA signal"=w475, "WA control switch"=w466, "WA signal switch"=w451, "WA extra"=w444) -> ()  [unwired: 8 in, 8 out]
  }
  n123 = disable-structure shown="Disabled" {
    frame #0 {
      # "Memory"
    }
    frame #1 {
    }
  }
  n124 = node-c288(w1) -> ()
  n125 = node-c288(w7) -> ()
